vi "Log_file_create_RIMAS.vi"(8 "error in (no error)":errorcluster, 10 "allow file creation":bool=TRUE, 11 "Mechanism name":string) -> (0 "error out":errorcluster, 2 "Current state  file name full":path, 3 "Log file name full":path, 4 "Created/existed?":bool, 5 "log file name":string caption="Log file name", 7 "Current state file name":string)   [LabVIEW 2021]
uses:
  Control - log directory.ctl
panel:
  in  "RIMAS log files path":T1=path "C:/RIMAS/logs" caption="start path"
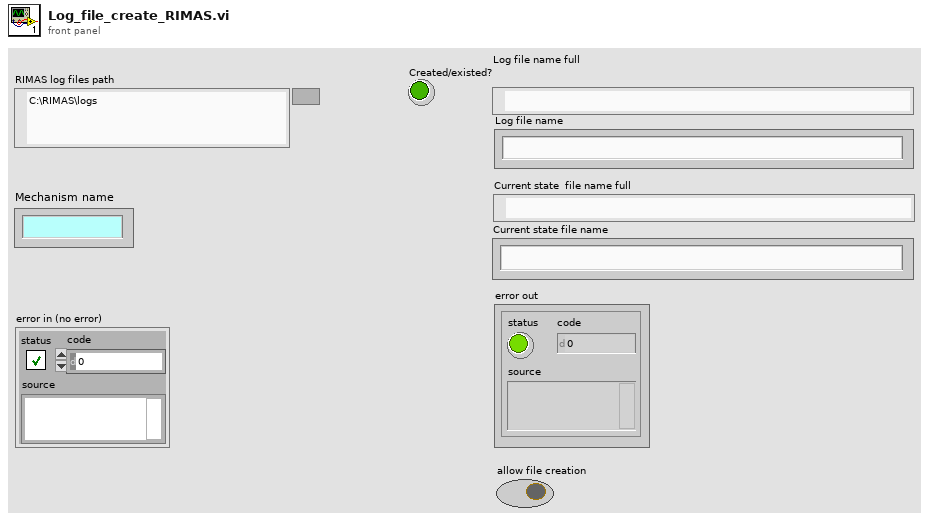
[diagram p1: front panel]
types:
  T1 = typedef "Control - log directory.ctl" = path
  T2 = enum16{"open", "replace", "create", "open or create", "replace or create", "replace or create with confirmation"}
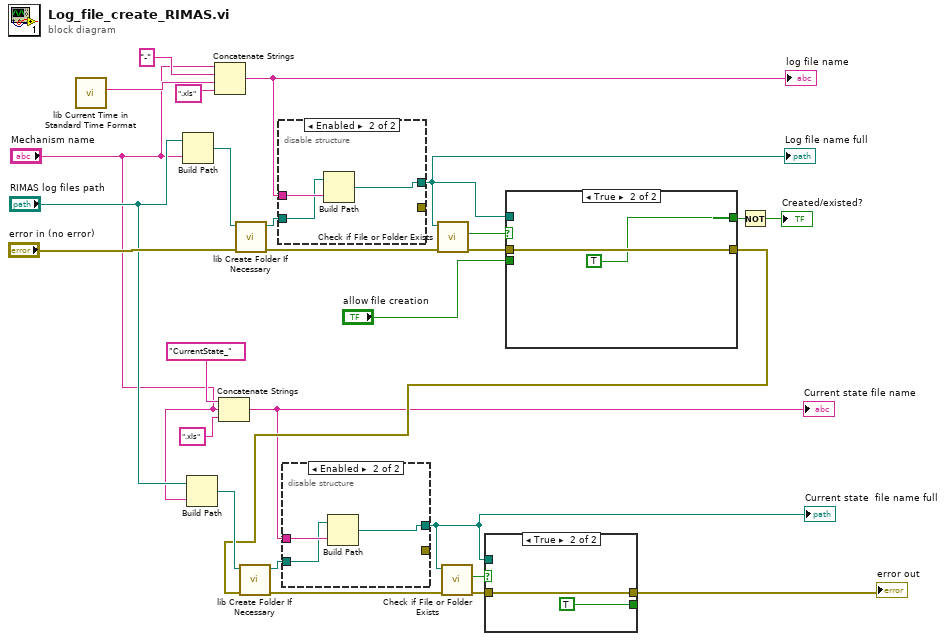
[diagram p0: block diagram]
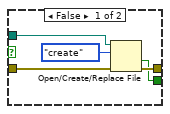
[diagram p2: hidden frame]
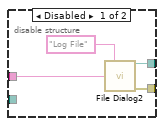
[diagram p3: hidden frame]
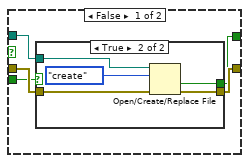
[diagram p4: hidden frame]
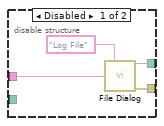
[diagram p6: hidden frame]
diagram:
  n1 = call "lib Current Time in Standard Time Format.vi"() -> ("date/time string"=w22:string)  [unwired: 11 in]
  n2 = Build Path(base path="RIMAS log files path", name or relative path="Mechanism name") -> (appended path=w26:path)
  n3 = Build Path(base path="RIMAS log files path", name or relative path="Mechanism name") -> (appended path=w13:path)
  n4 = Concatenate Strings("Mechanism name", "-", w22, ".xls" ("string")) -> (w25:string)
  "log file name" <- w25
  n5 = Concatenate Strings("CurrentState_", "Mechanism name", ".xls" ("string")) -> (w7:string)
  "Current state file name" <- w7
  n6 = call "lib Create Folder If Necessary.vi"("error in (no error)"="error in (no error)", "Folder"=w26) -> ("error out"=w19:errorcluster, "Folder dup"=w27:path)  [unwired: 8 in]
  n7 = disable-structure shown="Enabled" {
    disable-tunnel: w25 -> [w31 w34]
    disable-tunnel: [w30 w32] -> w24
    disable-tunnel: [w28 _] -> _
    disable-tunnel: w27 -> [_ w33]
    frame Disabled {
      n8 = call "File Dialog"("prompt"="Log File", "default name"=w31) -> ("selected path"=w30:path, "error out"=w28:errorcluster)  [unwired: 5 in, 7 out]
    }
    frame Enabled {
      n9 = Build Path(base path=w33, name or relative path=w34) -> (appended path=w32:path)
    }
  }
  "Log file name full" <- w24
  n10 = call <vilib>:"Check if File or Folder Exists.vi"("error in (no error)"=w19, "path"=w24) -> ("error out"=w18:errorcluster, "file or folder exists?"=w23:bool)  [unwired: 7 in, 1 out]
  n11 = case shown="True" w23 {
    tunnel: w18 -> [w39 w48]
    tunnel: w24 -> [w38 _]
    tunnel: [w37 w48] -> w10
    tunnel: [w36 TRUE ("cancelled")] -> w2
    tunnel: "allow file creation" -> [w35 _]
    frame False {
      n12 = case shown="True" w35 {
        selector: w35 -> [w40 _]
        tunnel: w39 -> [w41 w45]
        tunnel: w38 -> [_ w44]
        tunnel: [w41 w43] -> w37
        tunnel: [w40 w42] -> w36
        frame False {
        }
        frame True {
          n13 = Open/Create/Replace File(file path (use dialog)=w44, error in=w45, operation (0:open)=T2."create") -> (cancelled=w42:bool, error out=w43:errorcluster)  [unwired: 4 out]
        }
      }
    }
    frame True {
    }
  }
  n14 = call "lib Create Folder If Necessary.vi"("error in (no error)"=w10, "Folder"=w13) -> ("error out"=w15:errorcluster, "Folder dup"=w12:path)  [unwired: 8 in]
  n15 = disable-structure shown="Enabled" {
    disable-tunnel: w7 -> [w52 w55]
    disable-tunnel: [w51 w53] -> w6
    disable-tunnel: [w49 _] -> _
    disable-tunnel: w12 -> [_ w54]
    frame Disabled {
      n16 = call "File Dialog2"("prompt"="Log File", "default name"=w52) -> ("selected path"=w51:path, "error out"=w49:errorcluster)  [unwired: 5 in, 7 out]
    }
    frame Enabled {
      n17 = Build Path(base path=w54, name or relative path=w55) -> (appended path=w53:path)
    }
  }
  "Current state  file name full" <- w6
  n18 = call <vilib>:"Check if File or Folder Exists.vi"("error in (no error)"=w15, "path"=w6) -> ("error out"=w16:errorcluster, "file or folder exists?"=w14:bool)  [unwired: 7 in, 1 out]
  n19 = case shown="True" w14 {
    tunnel: w16 -> [w59 w62]
    tunnel: w6 -> [w58 _]
    tunnel: [w57 w62] -> w9
    tunnel: [w56 TRUE ("cancelled")] -> _
    frame False {
      n20 = Open/Create/Replace File(file path (use dialog)=w58, error in=w59, operation (0:open)=T2."create") -> (cancelled=w56:bool, error out=w57:errorcluster)  [unwired: 4 out]
    }
    frame True {
    }
  }
  "error out" <- w9
  n21 = Not(x=w2) -> (.not. x?=→"Created/existed?":bool)
